vi "Project.vi"() -> ()   [LabVIEW 2022 SP3]
uses:
  <vilib>/DAQmx/read.llb/DAQmx Read (Analog 1D DBL NChan 1Samp).vi
  <vilib>/DAQmx/write.llb/DAQmx Write (Digital Bool 1Line 1Point).vi
  <vilib>/DAQmx/create/channels.llb/DAQmx Create Channel (AI-Voltage-Basic).vi
  <vilib>/DAQmx/create/channels.llb/DAQmx Create Channel (DO-Digital Output).vi
  <vilib>/DAQmx/miscellaneous.llb/DAQmx Fill In Error Info.vi
panel:
  out "Real Time Variation of Gas Sensor Output":dbl(graph)
  in  "Buzzer for Gas Sensor":tag
  out "Real Time Temperature Variation":dbl(graph)
  in  "Fan Output":tag
  out "PIR Value":dbl
  out "Motion Detector":bool
  in  "Rain Sensor Output":tag
  out "Rain Sensor Value Indicator":dbl(knob) scale=0.0..6.0
  out "Rain Sensor Value":dbl
  in  "PIR Output for LED Lights":tag
  out "Voltage value":dbl
  out "Temp Value":dbl
  in  "Thermister Output for Buzzer":tag
  in  "stop 2":bool
  out "Temp Indicator":dbl(knob) scale=0.0..100.0
  out "Voltage":dbl(knob) scale=0.0..1.0
  in  "Sensor inputs":tag
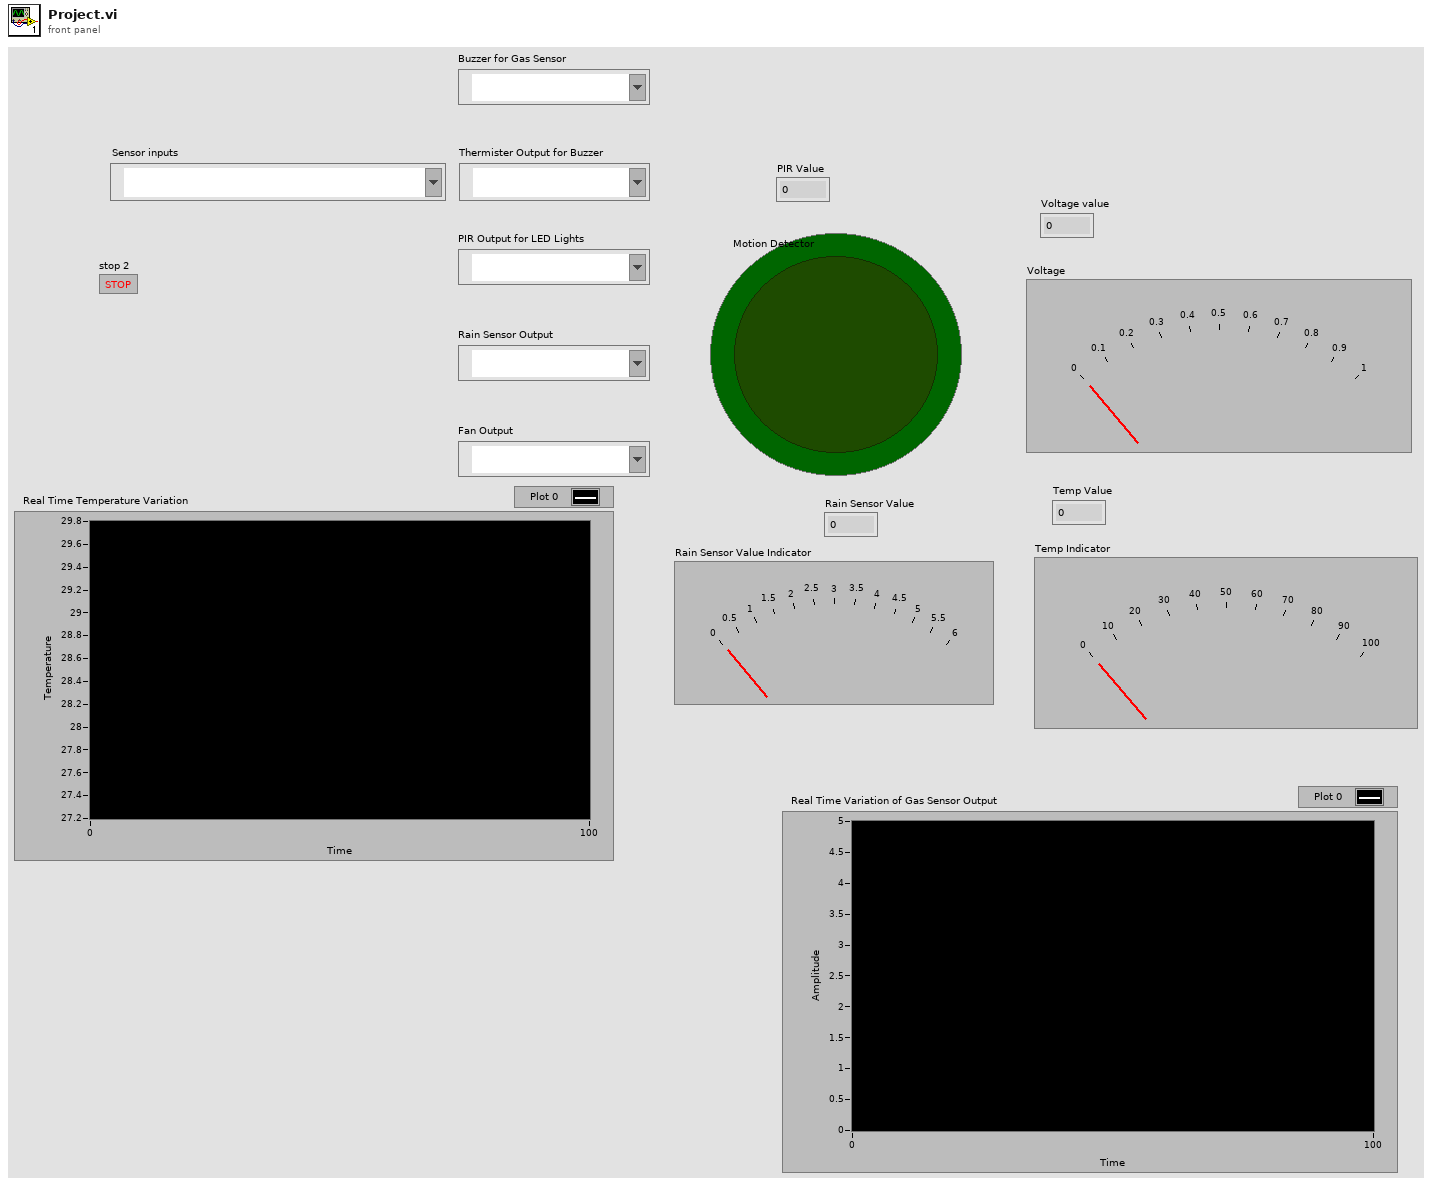
[diagram p1: front panel]
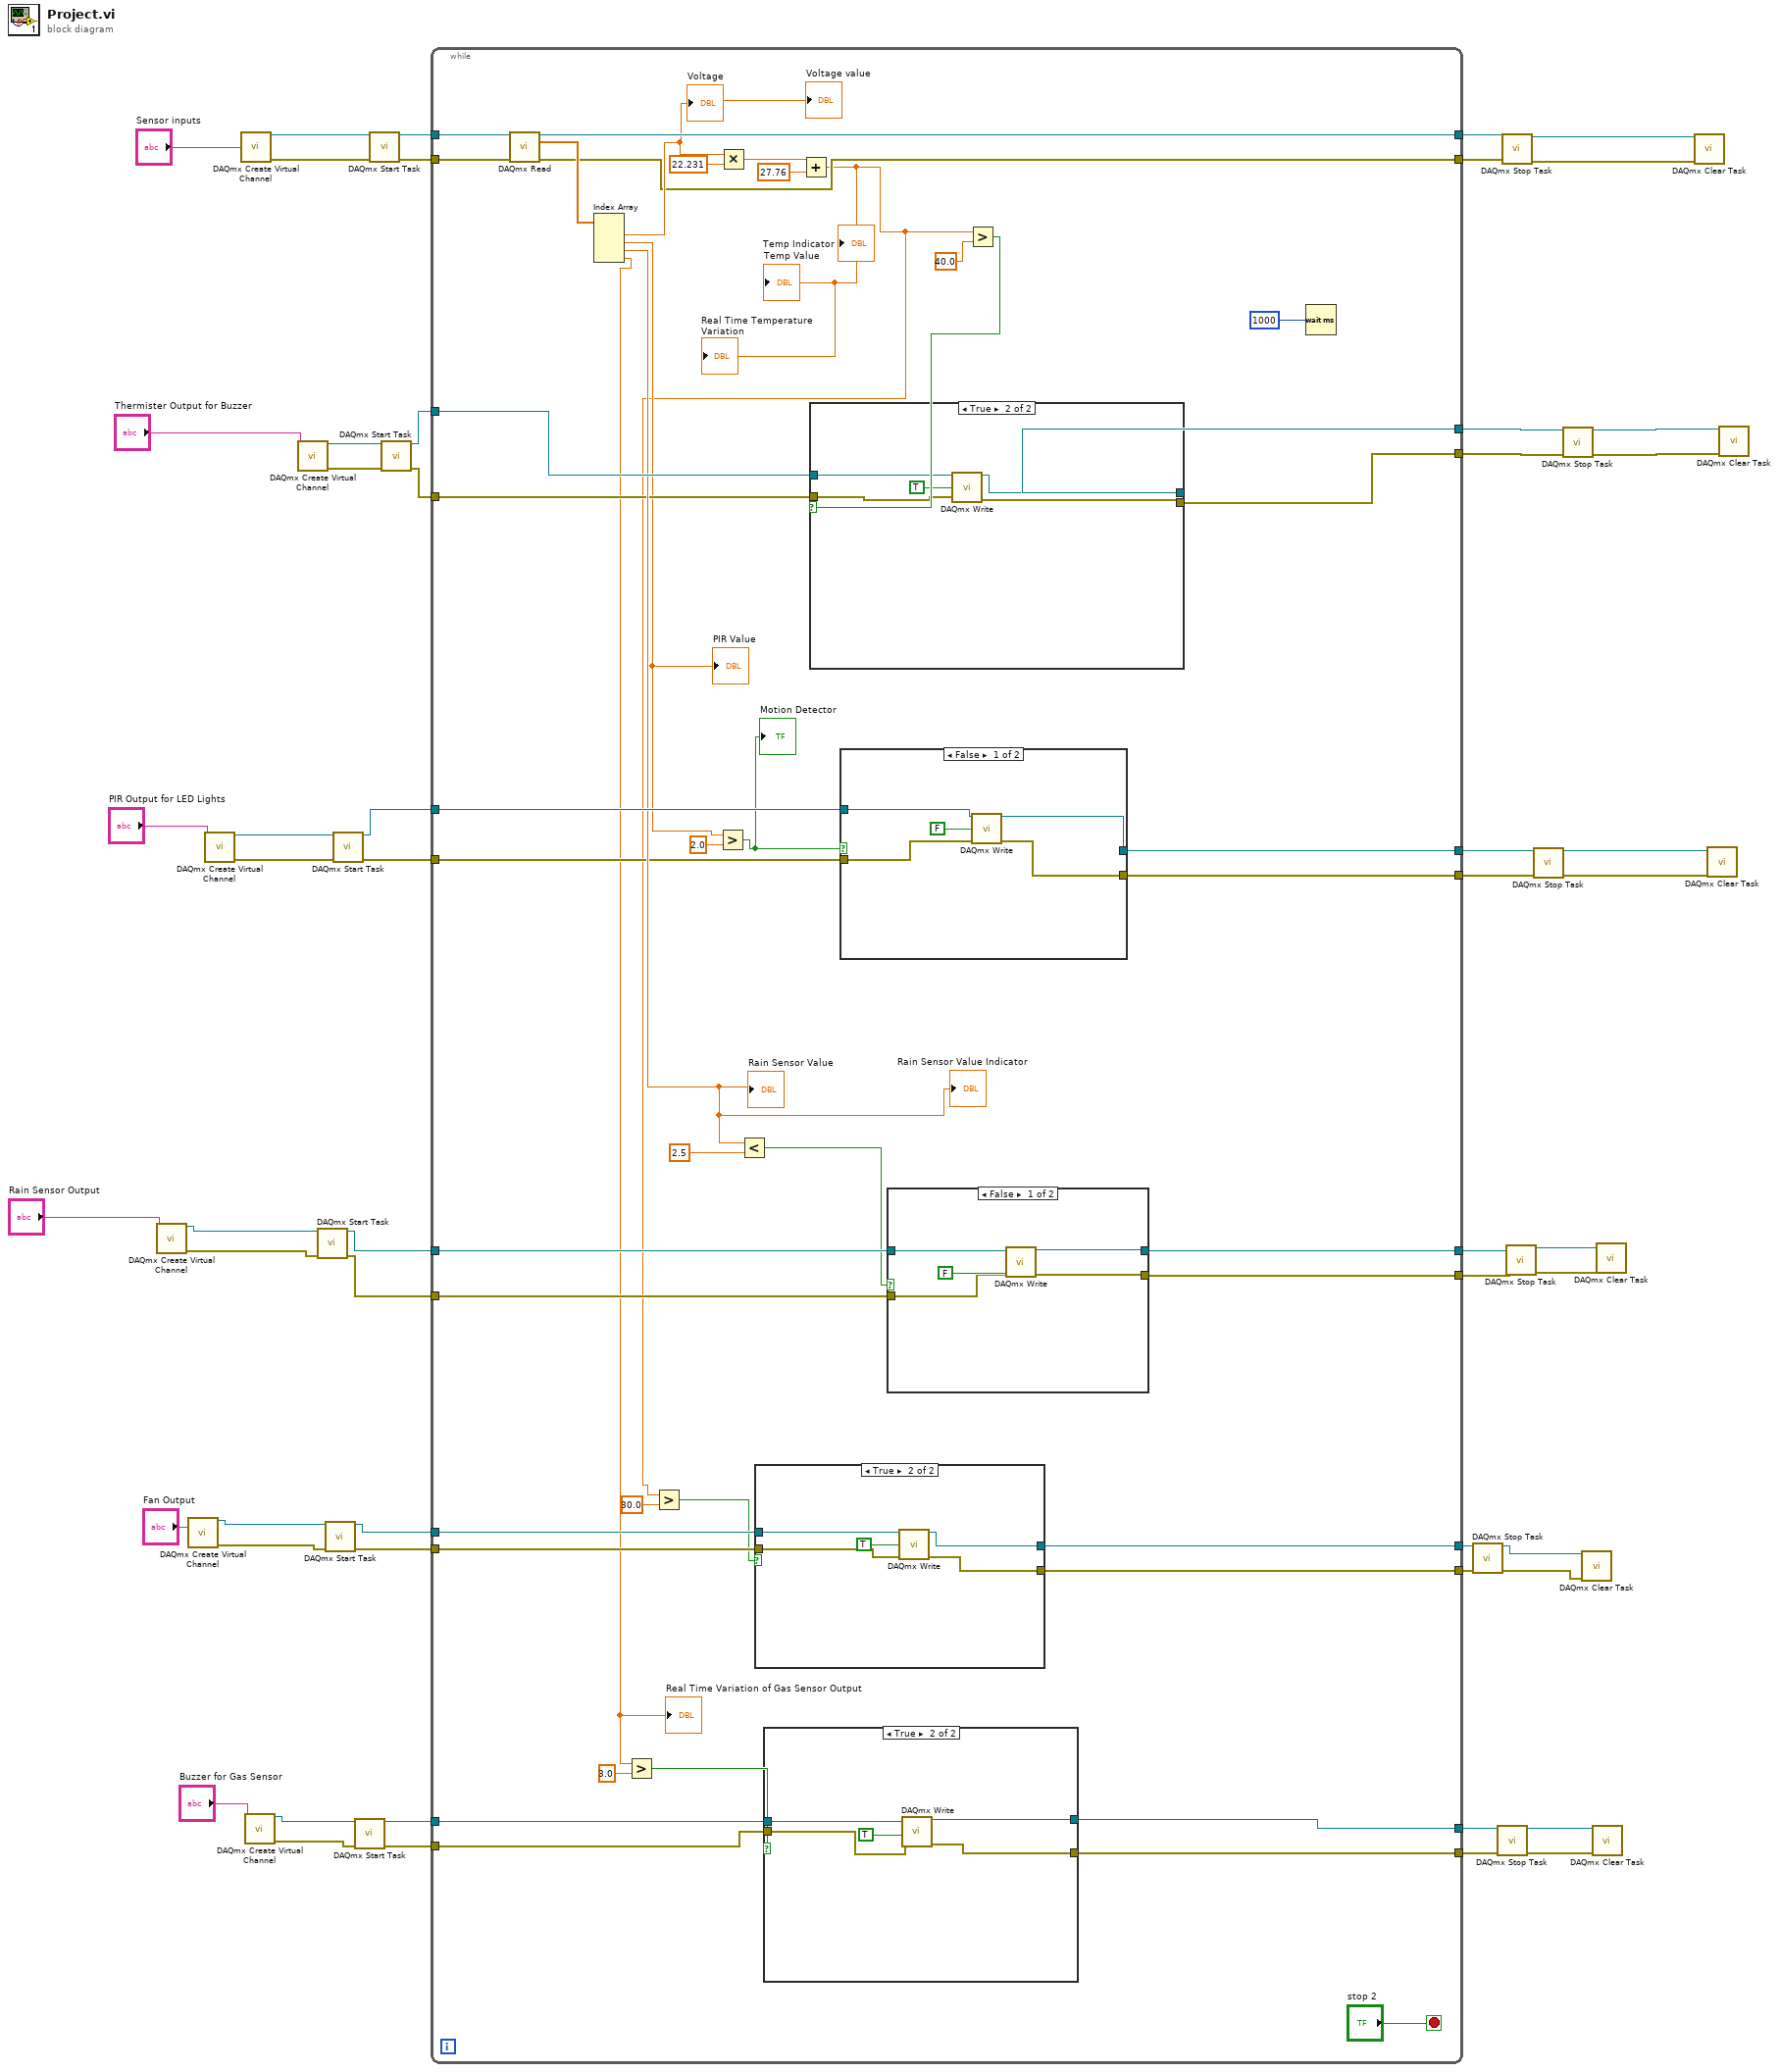
[diagram p0: block diagram]
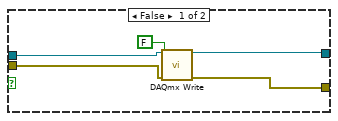
[diagram p2: hidden frame]
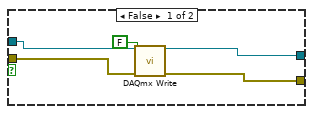
[diagram p3: hidden frame]
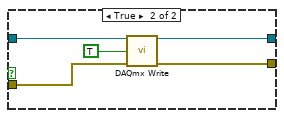
[diagram p4: hidden frame]
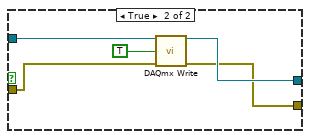
[diagram p5: hidden frame]
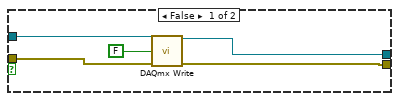
[diagram p6: hidden frame]
diagram:
  n1 = call-poly <vilib>:"DAQmx Create Virtual Channel.vi"("lines"="Rain Sensor Output") -> ("task out"=w38:refnum<k21>, "error out"=w22:errorcluster)  [unwired: 13 in]
  n2 = call-poly <vilib>:"DAQmx Create Virtual Channel.vi"("lines"="Fan Output") -> ("task out"=w18:refnum<k21>, "error out"=w14:errorcluster)  [unwired: 13 in]
  n3 = call-poly <vilib>:"DAQmx Create Virtual Channel.vi"("lines"="PIR Output for LED Lights") -> ("task out"=w43:refnum<k21>, "error out"=w26:errorcluster)  [unwired: 13 in]
  n4 = call-poly <vilib>:"DAQmx Create Virtual Channel.vi"("physical channels"="Sensor inputs") -> ("task out"=w53:refnum<k21>, "error out"=w34:errorcluster)  [unwired: 13 in]
  n5 = call-poly <vilib>:"DAQmx Create Virtual Channel.vi"("lines"="Buzzer for Gas Sensor") -> ("task out"=w8:refnum<k21>, "error out"=w4:errorcluster)  [unwired: 13 in]
  n6 = call-poly <vilib>:"DAQmx Create Virtual Channel.vi"("lines"="Thermister Output for Buzzer") -> ("task out"=w46:refnum<k21>, "error out"=w30:errorcluster)  [unwired: 13 in]
  n7 = call <vilib>:"DAQmx Start Task.vi"("task/channels in"=w38, "error in"=w22) -> ("task out"=w37:refnum<k21>, "error out"=w21:errorcluster)  [unwired: 12 in]
  n8 = call <vilib>:"DAQmx Start Task.vi"("task/channels in"=w18, "error in"=w14) -> ("task out"=w17:refnum<k21>, "error out"=w13:errorcluster)  [unwired: 12 in]
  n9 = call <vilib>:"DAQmx Start Task.vi"("task/channels in"=w43, "error in"=w26) -> ("task out"=w42:refnum<k21>, "error out"=w25:errorcluster)  [unwired: 12 in]
  n10 = call <vilib>:"DAQmx Start Task.vi"("task/channels in"=w8, "error in"=w4) -> ("task out"=w7:refnum<k21>, "error out"=w3:errorcluster)  [unwired: 12 in]
  n11 = call <vilib>:"DAQmx Start Task.vi"("task/channels in"=w53, "error in"=w34) -> ("task out"=w52:refnum<k21>, "error out"=w33:errorcluster)  [unwired: 12 in]
  n12 = call <vilib>:"DAQmx Start Task.vi"("task/channels in"=w46, "error in"=w30) -> ("task out"=w49:refnum<k21>, "error out"=w29:errorcluster)  [unwired: 12 in]
  n13 = while {
    tunnel: w52 -> [w99]
    tunnel: [w98] -> w50
    tunnel: w49 -> [w92]
    tunnel: [w91] -> w48
    tunnel: w42 -> [w88]
    tunnel: [w87] -> w41
    tunnel: w37 -> [w85]
    tunnel: [w83] -> w36
    tunnel: w33 -> [w79]
    tunnel: [w78] -> w32
    tunnel: w29 -> [w77]
    tunnel: [w76] -> w28
    tunnel: w25 -> [w75]
    tunnel: [w74] -> w24
    tunnel: w21 -> [w73]
    tunnel: [w72] -> w20
    tunnel: w17 -> [w68]
    tunnel: [w67] -> w16
    tunnel: w13 -> [w66]
    tunnel: [w65] -> w12
    tunnel: w7 -> [w61]
    tunnel: [w60] -> w6
    tunnel: w3 -> [w59]
    tunnel: [w58] -> w2
    stop <- "stop 2" stop-if-true
    n14 = call-poly <vilib>:"DAQmx Read.vi"("task/channels in"=w99, "error in"=w79) -> ("task out"=w98:refnum<k21>, "data"=w82:dbl[], "error out"=w78:errorcluster)  [unwired: 11 in]
    n15 = Index Array(array=w82) -> (element #1=w81:dbl, element #2=w69:dbl, element #3=w80:dbl, element #4=w55:dbl)  [unwired: 4 in]
    "Voltage" <- w81
    "Voltage value" <- w81
    "Rain Sensor Value" <- w80
    "Rain Sensor Value Indicator" <- w80
    "PIR Value" <- w69
    "Real Time Variation of Gas Sensor Output" <- w55
    n16 = Greater?(x=w55, y=3.0) -> (0:w56:bool)
    n17 = Greater?(x=w69, y=2.0) -> (0:w70:bool)
    "Motion Detector" <- w70
    n18 = Multiply(x=w81, y=22.231) -> (x*y=w96:dbl)
    n19 = Less?(x=w80, y=2.5) -> (x < y?=w84:bool)
    n20 = case shown="True" w56 {
      tunnel: w61 -> [w104 w108]
      tunnel: [w103 w107] -> w60
      tunnel: w59 -> [w102 w106]
      tunnel: [w101 w105] -> w58
      frame False {
        n21 = call-poly <vilib>:"DAQmx Write.vi"("task/channels in"=w104, "data"=FALSE, "error in"=w102) -> ("task out"=w103:refnum<k21>, "error out"=w101:errorcluster)  [unwired: 10 in, 1 out]
      }
      frame True {
        n22 = call-poly <vilib>:"DAQmx Write.vi"("task/channels in"=w108, "data"=TRUE, "error in"=w106) -> ("task out"=w107:refnum<k21>, "error out"=w105:errorcluster)  [unwired: 10 in, 1 out]
      }
    }
    n23 = Add(x=w96, y=27.76) -> (x+y=w62:dbl)
    "Temp Indicator" <- w62
    "Temp Value" <- w62
    "Real Time Temperature Variation" <- w62
    n24 = Greater?(x=w62, y=30.0) -> (0:w63:bool)
    n25 = case shown="True" w63 {
      tunnel: w68 -> [w114 w119]
      tunnel: [w113 w118] -> w67
      tunnel: w66 -> [w112 w117]
      tunnel: [w111 w116] -> w65
      frame False {
        n26 = call-poly <vilib>:"DAQmx Write.vi"("task/channels in"=w114, "data"=FALSE, "error in"=w112) -> ("task out"=w113:refnum<k21>, "error out"=w111:errorcluster)  [unwired: 10 in, 1 out]
      }
      frame True {
        n27 = call-poly <vilib>:"DAQmx Write.vi"("task/channels in"=w119, "data"=TRUE, "error in"=w117) -> ("task out"=w118:refnum<k21>, "error out"=w116:errorcluster)  [unwired: 10 in, 1 out]
      }
    }
    n28 = case shown="False" w70 {
      tunnel: w88 -> [w134 w138]
      tunnel: [w133 w137] -> w87
      tunnel: w75 -> [w131 w136]
      tunnel: [w130 w135] -> w74
      frame False {
        n29 = call-poly <vilib>:"DAQmx Write.vi"("task/channels in"=w134, "data"=FALSE, "error in"=w131) -> ("task out"=w133:refnum<k21>, "error out"=w130:errorcluster)  [unwired: 10 in, 1 out]
      }
      frame True {
        n30 = call-poly <vilib>:"DAQmx Write.vi"("task/channels in"=w138, "data"=TRUE, "error in"=w136) -> ("task out"=w137:refnum<k21>, "error out"=w135:errorcluster)  [unwired: 10 in, 1 out]
      }
    }
    n31 = case shown="False" w84 {
      tunnel: w85 -> [w123 w128]
      tunnel: [w122 w127] -> w83
      tunnel: w73 -> [w121 w126]
      tunnel: [w120 w125] -> w72
      frame False {
        n32 = call-poly <vilib>:"DAQmx Write.vi"("task/channels in"=w123, "data"=FALSE, "error in"=w121) -> ("task out"=w122:refnum<k21>, "error out"=w120:errorcluster)  [unwired: 10 in, 1 out]
      }
      frame True {
        n33 = call-poly <vilib>:"DAQmx Write.vi"("task/channels in"=w128, "data"=TRUE, "error in"=w126) -> ("task out"=w127:refnum<k21>, "error out"=w125:errorcluster)  [unwired: 10 in, 1 out]
      }
    }
    n34 = Greater?(x=w62, y=40.0) -> (0:w93:bool)
    n35 = case shown="True" w93 {
      tunnel: w92 -> [w142 w149]
      tunnel: [w143 w148] -> w91
      tunnel: w77 -> [w141 w146]
      tunnel: [w140 w145] -> w76
      frame False {
        n36 = call-poly <vilib>:"DAQmx Write.vi"("task/channels in"=w142, "data"=FALSE, "error in"=w141) -> ("task out"=w143:refnum<k21>, "error out"=w140:errorcluster)  [unwired: 10 in, 1 out]
      }
      frame True {
        n37 = call-poly <vilib>:"DAQmx Write.vi"("task/channels in"=w149, "data"=TRUE, "error in"=w146) -> ("task out"=w148:refnum<k21>, "error out"=w145:errorcluster)  [unwired: 10 in, 1 out]
      }
    }
    n38 = Wait (ms)(milliseconds to wait=u32 1000) -> ()  [unwired: 1 out]
  }
  n39 = call <vilib>:"DAQmx Stop Task.vi"("task/channels in"=w16, "error in"=w12) -> ("task out"=w15:refnum<k21>, "error out"=w11:errorcluster)  [unwired: 12 in]
  n40 = call <vilib>:"DAQmx Stop Task.vi"("task/channels in"=w6, "error in"=w2) -> ("task out"=w5:refnum<k21>, "error out"=w1:errorcluster)  [unwired: 12 in]
  n41 = call <vilib>:"DAQmx Stop Task.vi"("task/channels in"=w50, "error in"=w32) -> ("task out"=w51:refnum<k21>, "error out"=w31:errorcluster)  [unwired: 12 in]
  n42 = call <vilib>:"DAQmx Stop Task.vi"("task/channels in"=w36, "error in"=w20) -> ("task out"=w35:refnum<k21>, "error out"=w19:errorcluster)  [unwired: 12 in]
  n43 = call <vilib>:"DAQmx Stop Task.vi"("task/channels in"=w41, "error in"=w24) -> ("task out"=w40:refnum<k21>, "error out"=w23:errorcluster)  [unwired: 12 in]
  n44 = call <vilib>:"DAQmx Stop Task.vi"("task/channels in"=w48, "error in"=w28) -> ("task out"=w47:refnum<k21>, "error out"=w27:errorcluster)  [unwired: 12 in]
  n45 = call <vilib>:"DAQmx Clear Task.vi"("task in"=w15, "error in"=w11) -> ()  [unwired: 13 in, 1 out]
  n46 = call <vilib>:"DAQmx Clear Task.vi"("task in"=w5, "error in"=w1) -> ()  [unwired: 13 in, 1 out]
  n47 = call <vilib>:"DAQmx Clear Task.vi"("task in"=w35, "error in"=w19) -> ()  [unwired: 13 in, 1 out]
  n48 = call <vilib>:"DAQmx Clear Task.vi"("task in"=w51, "error in"=w31) -> ()  [unwired: 13 in, 1 out]
  n49 = call <vilib>:"DAQmx Clear Task.vi"("task in"=w40, "error in"=w23) -> ()  [unwired: 13 in, 1 out]
  n50 = call <vilib>:"DAQmx Clear Task.vi"("task in"=w47, "error in"=w27) -> ()  [unwired: 13 in, 1 out]
